vi "send image reference.vi"(8 "error in (no error)":errorcluster, 11 "DAQOrcaFlash in":refnum<class "DAQOrcaFlash.lvclass">) -> (0 "error out":errorcluster, 3 "DAQOrcaFlash out":refnum<class "DAQOrcaFlash.lvclass">)   [LabVIEW 2012, in "DAQOrcaFlash.lvclass"]
uses:
  DAQOrcaFlash.lvclass
  DAQOrcaFlash.lvclass/DAQOrcaFlash.ctl
  <vilib>/Distrio/Murmex/Murmex/Murmex.lvclass
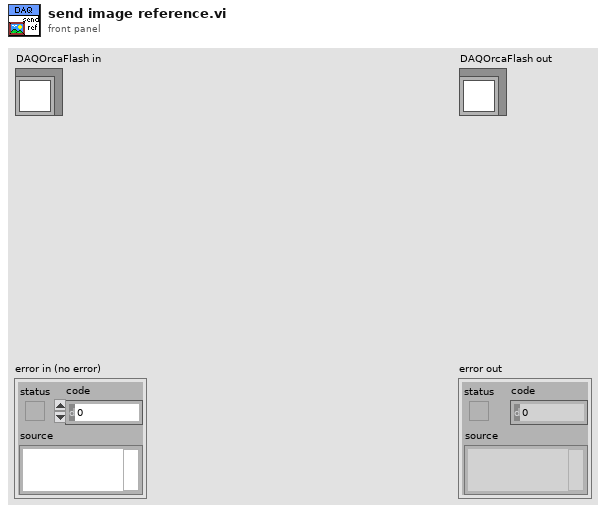
[diagram p1: front panel]
types:
  T1 = typedef "IMAQ Image.ctl" = refnum<image>
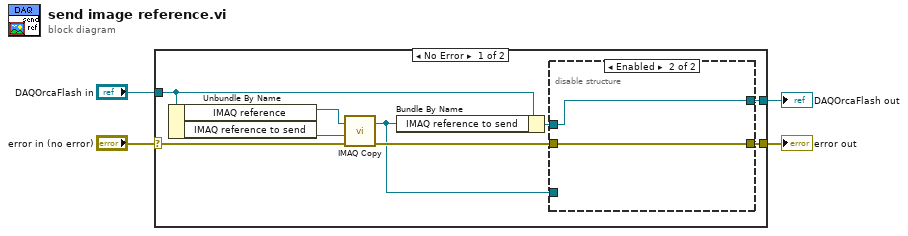
[diagram p0: block diagram]
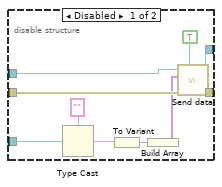
[diagram p2: hidden frame]
diagram:
  n1 = case shown="No Error" "error in (no error)" {
    selector: "error in (no error)" -> [w11 w27]
    tunnel: [w8 w27] -> w3
    tunnel: [w6 w26] -> w1
    tunnel: "DAQOrcaFlash in" -> [w10 w26]
    frame No Error {
      n2 = Unbundle By Name(w10) -> ("IMAQ reference"=w13:T1, "IMAQ reference to send"=w12:T1)
      n3 = call "IMAQ Copy"("error in (no error)"=w11, "Image Dst"=w12, "Image Src"=w13) -> ("error out"=w9:errorcluster, "Image Dst Out"=w5:T1)  [unwired: 3 in]
      n4 = Bundle By Name(cluster=w10, "IMAQ reference to send"=w5) -> (w7:refnum<class "DAQOrcaFlash.lvclass">)
      n5 = disable-structure shown="Enabled" {
        disable-tunnel: w9 -> [w22 w24]
        disable-tunnel: [w21 w24] -> w8
        disable-tunnel: w7 -> [w20 w25]
        disable-tunnel: [w19 w25] -> w6
        disable-tunnel: w5 -> [w16 _]
        frame Disabled {
          n6 = Type Cast(type="", x=w16) -> (*(type *) &x=w14:string)
          n7 = To Variant(anything=w14) -> (Variant=w23:variant)
          n8 = Build Array(w23) -> (w18:variant[])
          n9 = call <vilib>:"Send data.vi"("is finalised data? (T)"=TRUE, "error in (no error)"=w22, "data (channels array)"=w18, "Murmex in"=w20) -> ("error out"=w21:errorcluster, "Murmex out"=w19:refnum<class "DAQOrcaFlash.lvclass">)  [unwired: 6 in]
        }
        frame Enabled {
        }
      }
    }
    frame Error {
    }
  }
  "error out" <- w3
  "DAQOrcaFlash out" <- w1
